vi "Switch.vi"(1 "In":bool) -> (0 "out":bool)   [LabVIEW 2013]
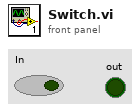
[diagram p1: front panel]
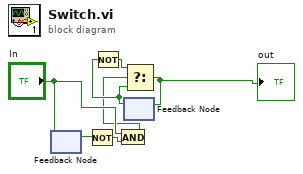
[diagram p0: block diagram]
diagram:
  n1 = feedback #1() -> (w4:bool)  [unwired: 1 in]
  n2 = feedback-in #1("In") -> ()
  n3 = Not(x=w4) -> (.not. x?=w3:bool)
  n4 = And(x="In", y=w3) -> (x .and. y?=w1:bool)
  n5 = feedback #2() -> (w5:bool)  [unwired: 1 in]
  n6 = Not(x=w5) -> (.not. x?=w6:bool)
  n7 = Select(t=w6, s=w1, f=w5) -> (s? t:f=w7:bool)
  "out" <- w7
  n8 = feedback-in #2(w7) -> ()
